vi "Group Delay.vi"() -> ()   [LabVIEW 2023]
doc: "This example shows how to obtain the group delay of a filter with the TFA Group Delay VI. \n\n<b>Requirements:</b>\nThis example requires the NI LabVIEW Digital Filter Design Toolkit.\n\n<b>Instructions:</b>\nRun this VI to observe group delays from the TFA method and DFD method."
uses:
  <vilib>/Analysis/baseanly.llb/IIR Cascade Filter (DBL).vi
  <vilib>/addons/Time Frequency Analysis/Spectrogram.llb/TFA STFT Spectrogram (Real).vi
  <vilib>/addons/Time Frequency Analysis/_control.llb/TFA Configure Spectrogram Indicator (Predefined Color Table).vi
  <vilib>/addons/_Advanced Signal Processing/NI_AdvSigProcTFA.lvlib
  <vilib>/Analysis/NI_AALBase.lvlib
  <vilib>/addons/Digital Filter Design/NI_DigFilterLicensed.lvlib
panel:
  out "aspt-left-top":bool
  out "Spectrogram of the Impulse Response":dbl[][](graph)
  out "Impulse Response":dbl[](graph)
  in  "Low cutoff frequency":dbl=0.30000000000000004 min=0.0 max=0.5 step=0.1
  out "Group Delay of the Filter":cluster{"f0":dbl, "df":dbl, "values":dbl[]}[](graph)
  in  "Order":i32=2
  # "Overview: Shows how to obtain the group delay of a filter with the TFA Group Delay VI. \nRequirements: LabVIEW Full Development System, Advanced Signal Processing Toolkit, Digital Filter Design Toolkit\nInstructions: \nRun this VI to observe group delays from the TFA method and DFD method."
  # "Filter Specification"
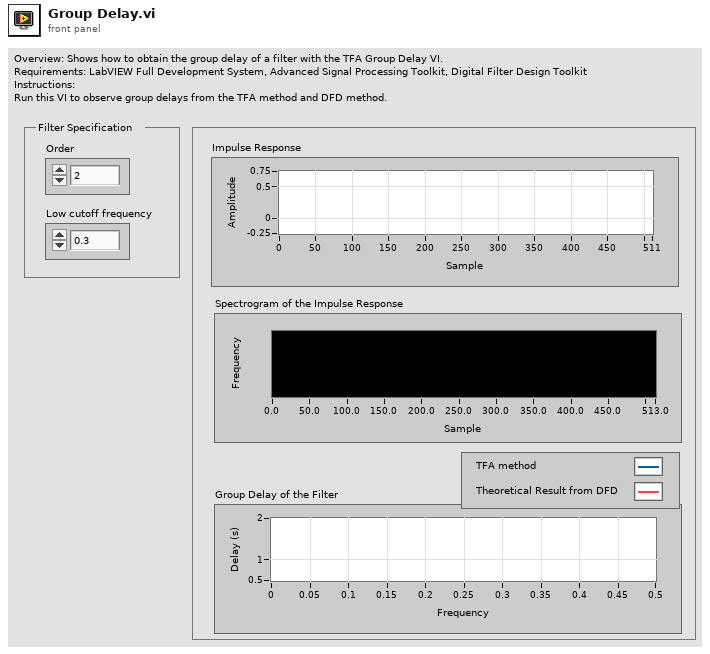
[diagram p1: front panel]
types:
  T1 = cluster{"filter structure":enum32{"IIR 2nd Order", "IIR 4th Order"}, "Reverse Coefficients":dbl[], "Forward Coefficients":dbl[]}
  T2 = typedef "NI_DigFilterLicensed.lvlib/DFD Filter Obj.ctl" = cluster{"mSRate_Fs":dbl, "mSRate_Version":string, "mSRate_Comments":string, "mSRate_OrgCoef":T3, "mSRate_CurCoef":T3, "mSRate_Quantized?":bool, "mSRate_QCoef":T3, "mSRate_QSettings":T5[], "mSRate_Order":i32, "mSRate_Scaling":cluster{"mSRate_ScaleByPowerOf2?":bool, "mSRate_ScaleType":T7}}
  T3 = typedef "NI_DigFilterLicensed.lvlib/DFD Filter Coef.ctl" = cluster{"type":T4, "gain":dbl, "coef a (k)":dbl[], "coef b (v)":dbl[]}
  T4 = typedef "NI_DigFilterLicensed.lvlib/DFD Filter Structure Type Selector.ctl" = enum16{"Undefined", "FIR Direct Form", "FIR Direct Form Transposed", "FIR Symmetric", "FIR Antisymmetric", "IIR Direct Form I", "IIR Direct Form I Transposed", "IIR Direct Form II", "IIR Direct Form II Transposed", "IIR Cascaded Second Order Sections Form I", "IIR Cascaded Second Order Sections Form I Transposed", "IIR Cascaded Second Order Sections Form II", "IIR Cascaded Second Order Sections Form II Transposed", "Lattice Allpass (basic sections)", "Lattice Allpass (one multiplier sections)", "Lattice Allpass (normalized sections)", "Lattice AR (basic sections)", "Lattice AR (one multiplier sections)", "Lattice AR (normalized sections)", "Lattice MA (minimum phase)", "Lattice MA (maximum phase)", "Lattice ARMA (basic sections)", "Lattice ARMA (one multiplier sections)", "Lattice ARMA (normalized sections)"}
  T5 = typedef "NI_DigFilterLicensed.lvlib/dfd_Internal Quantization Settings.ctl" = cluster{"source":T6, "wl":i16, "iwl":i16, "overflow mode":enum16{"Saturation", "Wrap"}, "rounding mode":enum16{"Nearest", "Truncation"}, "signed?":bool}
  T6 = typedef "NI_DigFilterLicensed.lvlib/dfd_Internal Quantization Srcs.ctl" = u16
  T7 = typedef "NI_DigFilterLicensed.lvlib/DFD Coef Norm Type.ctl" = enum16{"No Norm", "Time Domain 1-Norm", "Time Domain 2-Norm", "Time Domain Inf-Norm"}
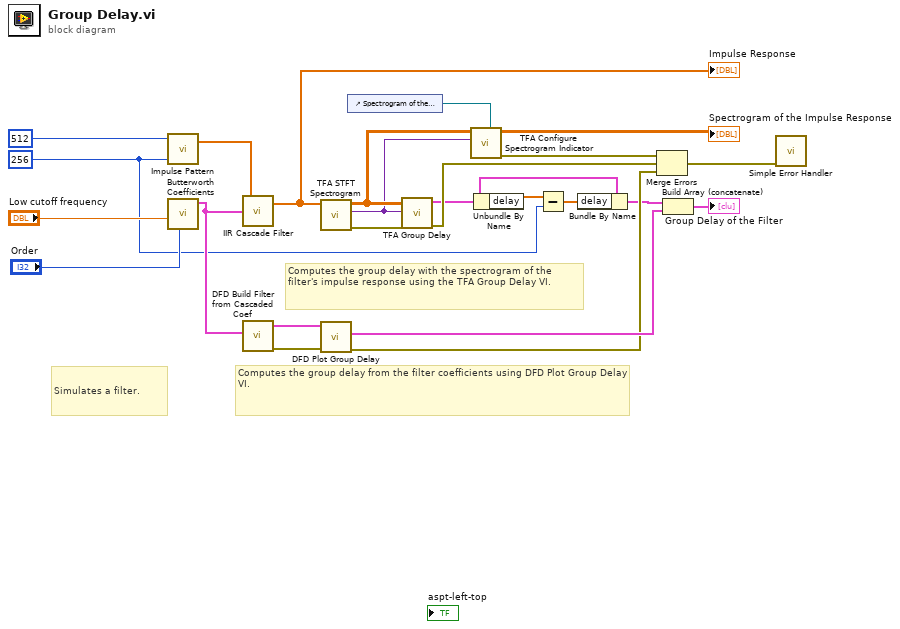
[diagram p0: block diagram]
diagram:
  w10 = 256 ("delay")
  # "Computes the group delay from the filter coefficients using DFD Plot Group Delay VI."
  # "Computes the group delay with the spectrogram of the filter's impulse response using the TFA Group Delay VI."
  # "Simulates a filter."
  n1 = call <vilib>:"Impulse Pattern.vi"("delay"=w10, "samples"=512) -> ("Impulse Pattern"=w16:dbl[])  [unwired: 1 in, 1 out]
  n2 = call <vilib>:"Butterworth Coefficients.vi"("order"="Order", "low cutoff freq: fl"="Low cutoff frequency") -> ("IIR Filter Cluster"=w15:T1)  [unwired: 8 in, 1 out]
  n3 = call-poly <vilib>:"IIR Cascade Filter.vi"("IIR Filter Cluster"=w15, "X"=w16) -> ("Filtered X"=w17:dbl[])  [unwired: 1 in, 1 out]
  "Impulse Response" <- w17
  n4 = call <vilib>:"DFD Build Filter from Cascaded Coef.vi"("IIR Filter Cluster"=w15) -> ("error out"=w13:errorcluster, "filter out"=w14:T2)  [unwired: 2 in, 7 out]
  n5 = call-poly <vilib>:"TFA STFT Spectrogram.vi"("signal"=w17) -> ("error out"=w9:errorcluster, "scale info"=w19:variant, "spectrogram"=w20:dbl[][])  [unwired: 3 in, 5 out]
  n6 = call <vilib>:"DFD Plot Group Delay.vi"("error in (no error)"=w13, "filter in"=w14) -> ("error out"=w6:errorcluster, "group delay"=w11:cluster{"f0":dbl, "df":dbl, "values":dbl[]}[])  [unwired: 2 in, 6 out]
  n7 = control-ref of="Spectrogram of the Impulse Response"() -> (w21:refnum<vi>)
  n8 = call <vilib>:"TFA Group Delay.vi"("error in (no error)"=w9, "scale info"=w19, "spectrogram"=w20) -> ("error out"=w7:errorcluster, "group delay"=w4:cluster{"f0":dbl, "df":dbl, "delay":dbl[]})  [unwired: 7 out]
  n9 = call-poly <vilib>:"TFA Configure Spectrogram Indicator.vi"("reference of TF spectrogram indicator"=w21, "scale info"=w19, "spectrogram"=w20) -> ("error out"=w8:errorcluster, "TF spectrogram indicator"=→"Spectrogram of the Impulse Response":dbl[][])  [unwired: 4 in, 3 out]
  n10 = Unbundle By Name(w4) -> ("delay"=w2:dbl[])
  n11 = Subtract(x=w2, y=w10) -> (x-y=w1:dbl[])
  n12 = Bundle By Name(cluster=w4, "delay"=w1) -> (w3:cluster{"f0":dbl, "df":dbl, "delay":dbl[]})
  n13 = Merge Errors(w8, w7, w6) -> (w5:errorcluster)
  n14 = Build Array (concatenate)(w3, w11) -> (→"Group Delay of the Filter":cluster{"f0":dbl, "df":dbl, "values":dbl[]}[])
  n15 = call <vilib>:"Simple Error Handler.vi"("error in (no error)"=w5) -> ()  [unwired: 4 in, 5 out]
